vi "Default Object.vi"() -> (2 "Actor":refnum<class "Actor.lvclass">)   [LabVIEW 2025, in "jettl.lvlib" / "Core Actor.lvlib"]
uses:
  Core Actor.lvlib
  Actor/Actor.lvclass
  Core Actor/Core Actor.lvclass
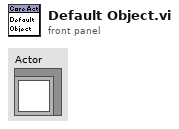
[diagram p1: front panel]
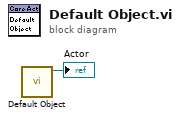
[diagram p0: block diagram]
diagram:
  n1 = call "Default Object.vi"() -> ("Core Actor out"=→"Actor":refnum<class "Core Actor.lvclass">)  [unwired: 11 in]
